vi "PhotonCamera_SetDriverMode.vi"(9 "DriverMode":bool, 11 "CameraName":string) -> ()   [LabVIEW 2019, in "PhotonVisionLib.lvlib"]
doc: "Toggles driver mode.\n \nInputs:\n - cameraName -- The nickname of the camera (found in the PhotonVision UI).\n - DriverMode -- Whether to set driver mode.\nOutputs:\n - >none<"
uses:
  PhotonVisionLib.lvlib
  <vilib>/Rock Robotics/Network Tables/NT Write Boolean.vi
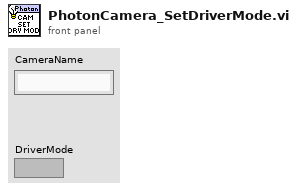
[diagram p1: front panel]
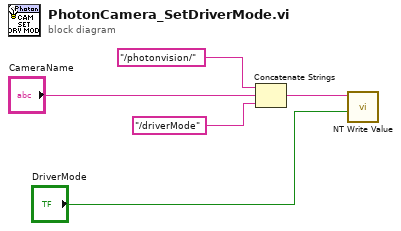
[diagram p0: block diagram]
diagram:
  n1 = Concatenate Strings("/photonvision/", "CameraName", "/driverMode") -> (w2:string)
  n2 = call-poly <vilib>:"NT Write Value.vi"("Boolean"="DriverMode", "Name"=w2) -> ()  [unwired: 9 in, 1 out]
